vi "Get Data.vi"(8 "error in (no error)":errorcluster, 10 "Number of samples":i32=-1, 11 "DAQmx Digitizer in":refnum<class "DAQmx Digitizer.lvclass">) -> (0 "error out":errorcluster, 3 "DAQmx Digitizer out":refnum<class "DAQmx Digitizer.lvclass">)   [LabVIEW 2015, in "DAQmx Digitizer.lvclass"]
uses:
  DAQmx Digitizer.lvclass
  DAQmx Digitizer.lvclass/DAQmx Digitizer.ctl
  <vilib>/DAQmx/read.llb/DAQmx Read (Analog 2D I16 NChan NSamp).vi
  <vilib>/DAQmx/miscellaneous.llb/DAQmx Fill In Error Info.vi
  <resource>/objmgr/daqmx.rc
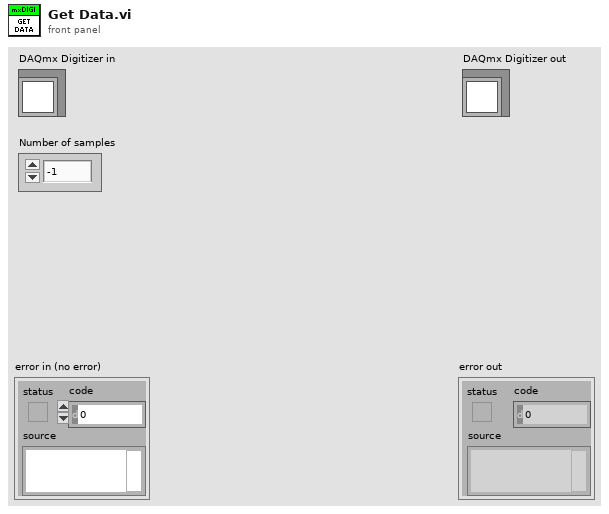
[diagram p1: front panel]
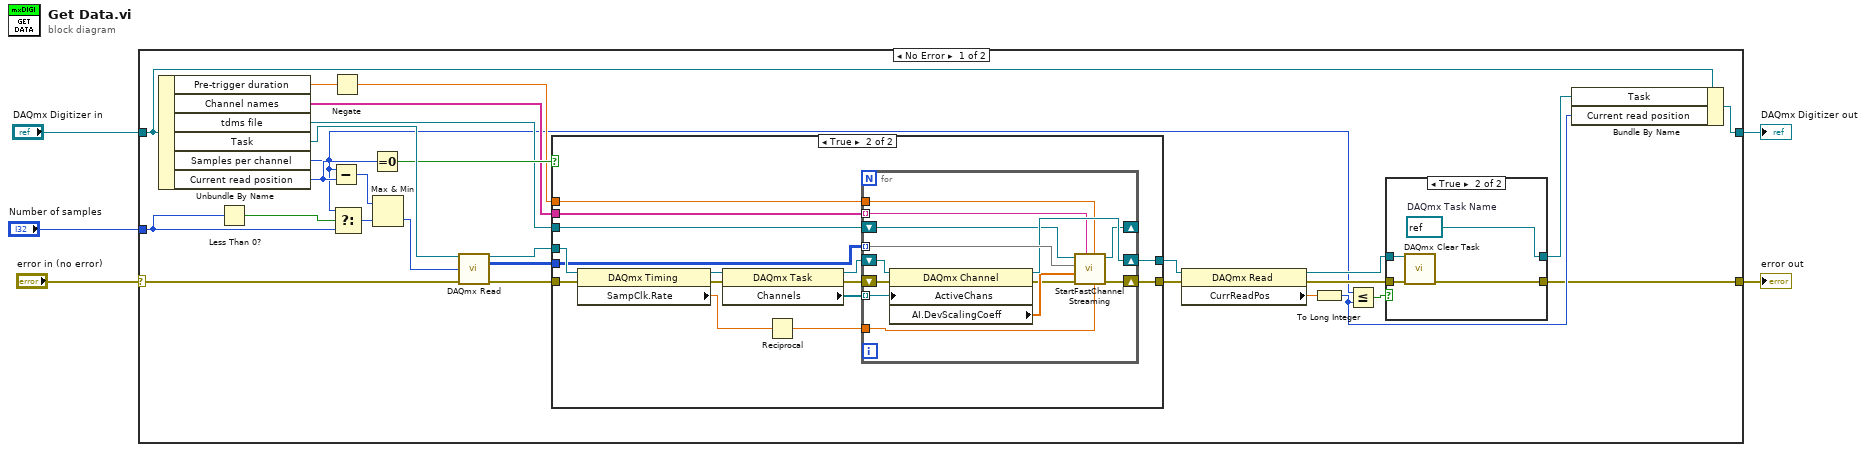
[diagram p0: block diagram]
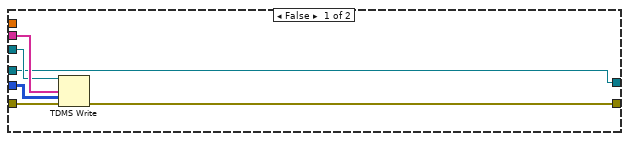
[diagram p3: hidden frame]
diagram:
  n1 = case shown="No Error" "error in (no error)" {
    selector: "error in (no error)" -> [w20 w75]
    tunnel: [w10 w75] -> w4
    tunnel: [w19 w74] -> w2
    tunnel: "DAQmx Digitizer in" -> [w33 w74]
    tunnel: "Number of samples" -> [w7 _]
    frame No Error {
      n2 = Unbundle By Name(w33) -> ("Pre-trigger duration"=w23:dbl, "Channel names"=w22:string[], "tdms file"=w21:refnum<k34>, "Task"=w31:refnum<k21>, "Samples per channel"=w8:i32, "Current read position"=w27:i32)
      n3 = Less Than 0?(x=w7) -> (x < 0?=w9:bool)
      n4 = Subtract(x=w8, y=w27) -> (x-y=w32:i32)
      n5 = Negate(x=w23) -> (-x=w24:dbl)
      n6 = Select(t=w8, s=w9, f=w7) -> (s? t:f=w6:i32)
      n7 = Equal To 0?(x=w27) -> (x = 0?=w26:bool)
      n8 = Max & Min(x=w32, y=w6) -> (min(x,y)=w30:i32)  [unwired: 1 out]
      n9 = call-poly <vilib>:"DAQmx Read.vi"("task/channels in"=w31, "number of samples per channel"=w30, "error in"=w20) -> ("task out"=w29:refnum<k21>, "data"=w25:i16[][], "error out"=w28:errorcluster)  [unwired: 1 in, 9 out]
      n10 = case shown="True" w26 {
        tunnel: w29 -> [w40 w60]
        tunnel: w28 -> [w42 w59]
        tunnel: w25 -> [w45 w58]
        tunnel: w24 -> [_ w53]
        tunnel: w22 -> [w44 w52]
        tunnel: w21 -> [w43 w51]
        tunnel: [w41 w48] -> w18
        tunnel: [w40 w47] -> w17
        frame False {
          n11 = TDMS Write(0:w43, 7:w44, 9:w45, 11:w42) -> (15:w41:errorcluster)  [unwired: 2 in, 3 out]
        }
        frame True {
          n12 = property class="DAQmx Timing"(reference=w60, error in=w59) -> (reference out=w56:refnum<k21>, error out=w57:errorcluster, "SampClk.Rate"=w55:dbl)
          n13 = property class="DAQmx Task"(reference=w56, error in=w57) -> (reference out=w49:refnum<k21>, error out=w50:errorcluster, "Channels"=w46:refnum<k21>[])
          n14 = Reciprocal(x=w55) -> (1/x=w54:dbl)
          n15 = for {
            tunnel: w58 -> [w73] mode=indexing
            shift-right: [w71] -> w47
            shift-left: w49 -> [w72]
            tunnel: w54 -> [w69]
            tunnel: w53 -> [w68]
            tunnel: w52 -> [w67] mode=indexing
            shift-right: [w65] -> _
            shift-left: w51 -> [w66]
            shift-right: [w62] -> w48
            shift-left: w50 -> [w64]
            tunnel: w46 -> [w61] mode=indexing
            n16 = property class="DAQmx Channel"(reference=w72, error in=w64, "ActiveChans"=w61) -> (reference out=w71:refnum<k21>, error out=w63:errorcluster, "AI.DevScalingCoeff"=w70:dbl[])
            n17 = call "StartFastChannelStreaming.vi"("dt"=w69, "t0"=w68, "channel name(s) in (Untitled)"=w67, "error in (no error)"=w63, "Scaling coefficients"=w70, "Data"=w73, "tdms file"=w66) -> ("error out"=w62:errorcluster, "tdms file out"=w65:refnum<k34>)  [unwired: 3 in]
          }
        }
      }
      n18 = property class="DAQmx Read"(reference=w17, error in=w18) -> (reference out=w12:refnum<k21>, error out=w13:errorcluster, "CurrReadPos"=w16:dbl)
      n19 = To Long Integer(number=w16) -> (32bit integer=w15:i32)
      n20 = Less Or Equal?(x=w8, y=w15) -> (x <= y?=w14:bool)
      n21 = case shown="True" w14 {
        tunnel: [w35 w39] -> w10
        tunnel: w12 -> [w34 w37]
        tunnel: w13 -> [w35 w38]
        tunnel: [w34 w36] -> w11
        frame False {
        }
        frame True {
          w36 = refnum<k21> refnum  # DAQmx Task Name
          n22 = call <vilib>:"DAQmx Clear Task.vi"("task in"=w37, "error in"=w38) -> ("error out"=w39:errorcluster)  [unwired: 13 out]
        }
      }
      n23 = Bundle By Name(cluster=w33, "Task"=w11, "Current read position"=w15) -> (w19:refnum<class "DAQmx Digitizer.lvclass">)
    }
    frame Error {
    }
  }
  "error out" <- w4
  "DAQmx Digitizer out" <- w2
